vi "FTW-TestSupport-Reflection-TypeCoverage.vi"(0 "Types Tested":T1[](array[typedef]), 5 "Skip Types that cannot be instantiated":bool=TRUE, 11 "error in":errorcluster) -> (15 "error out":errorcluster)   [LabVIEW 2014]
uses:
  src/reflection/FTW-Reflection-Types.ctl
  src/error/FTW-ERR-ThrowError.vi
  src/error/FTW-ERR-NoErrorConstant.vi
  src/error/FTW-ERR-CallChain.vi
  src/string/FTW-STR-ReplaceWhitespace.vi
panel:
  # "Inputs"
  # "Outputs"
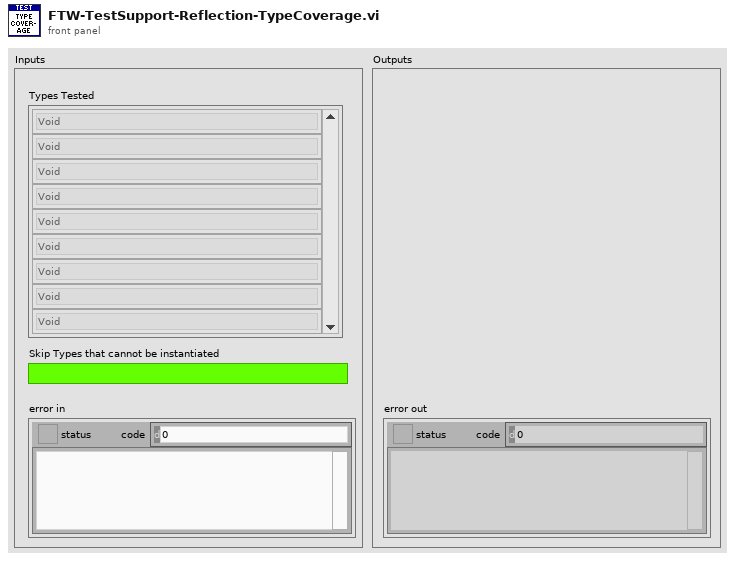
[diagram p1: front panel]
types:
  T1 = typedef "FTW-Reflection-Types.ctl" = enum16{"Unknown", "Void", "Array", "Cluster", "LVObject", "Boolean", "I8", "I16", "I32", "I64", "U8", "U16", "U32", "U64", "SGL", "DBL", "EXT", "CSG", "CDB", "CXT", "FXP", "EnumU8", "EnumU16", "EnumU32", "EnumU64", "SGLwithUnit", "DBLwithUnit", "EXTwithUnit", "CSGwithUnit", "CDBwithUnit", "CXTwithUnit", "String", "Path", "Picture", "Tag", "LVVariant", "Timestamp", "WaveformI8", "WaveformI16", "WaveformI32", "WaveformI64", "WaveformU8", "WaveformU16", "WaveformU32", "WaveformU64", "WaveformSGL", "WaveformDBL", "WaveformEXT", "WaveformCSG", "WaveformCDB", "WaveformCXT", "WaveformDigital", "WaveformUnknownType", "DigitalData", "DynamicData", "ExternalData", "FileByteStream", "TDMStream", "dotNET", "ActiveX", "VIServerReference", "VIReference", "ApplicationInstance", "Menu", "ConnectionDataSocket", "ConnectionVISA", "ConnectionBluetooth", "ConnectionIrDA", "ConnectionTCP", "ConnectionUDP", "ConnectionHTTPClient", "ConnectionFTP", "Occurrence", "Notifier", "Queue", "Rendezvous", "Semaphore", "RTFIFO", "EventPublisher", "EventRegistration", "EventCallback", "DataValueReference", "GenericClass", "GenericClassTag", "GenericClassDeepCopy", "GenericClassFlattened", "GenericClassTagFlattened", "GenericReferenceType", "WindowsRegistry", "OverloadedDatalogRef", "ReferenceUnknownType", "ByteArray", "ConPaneInterface"}
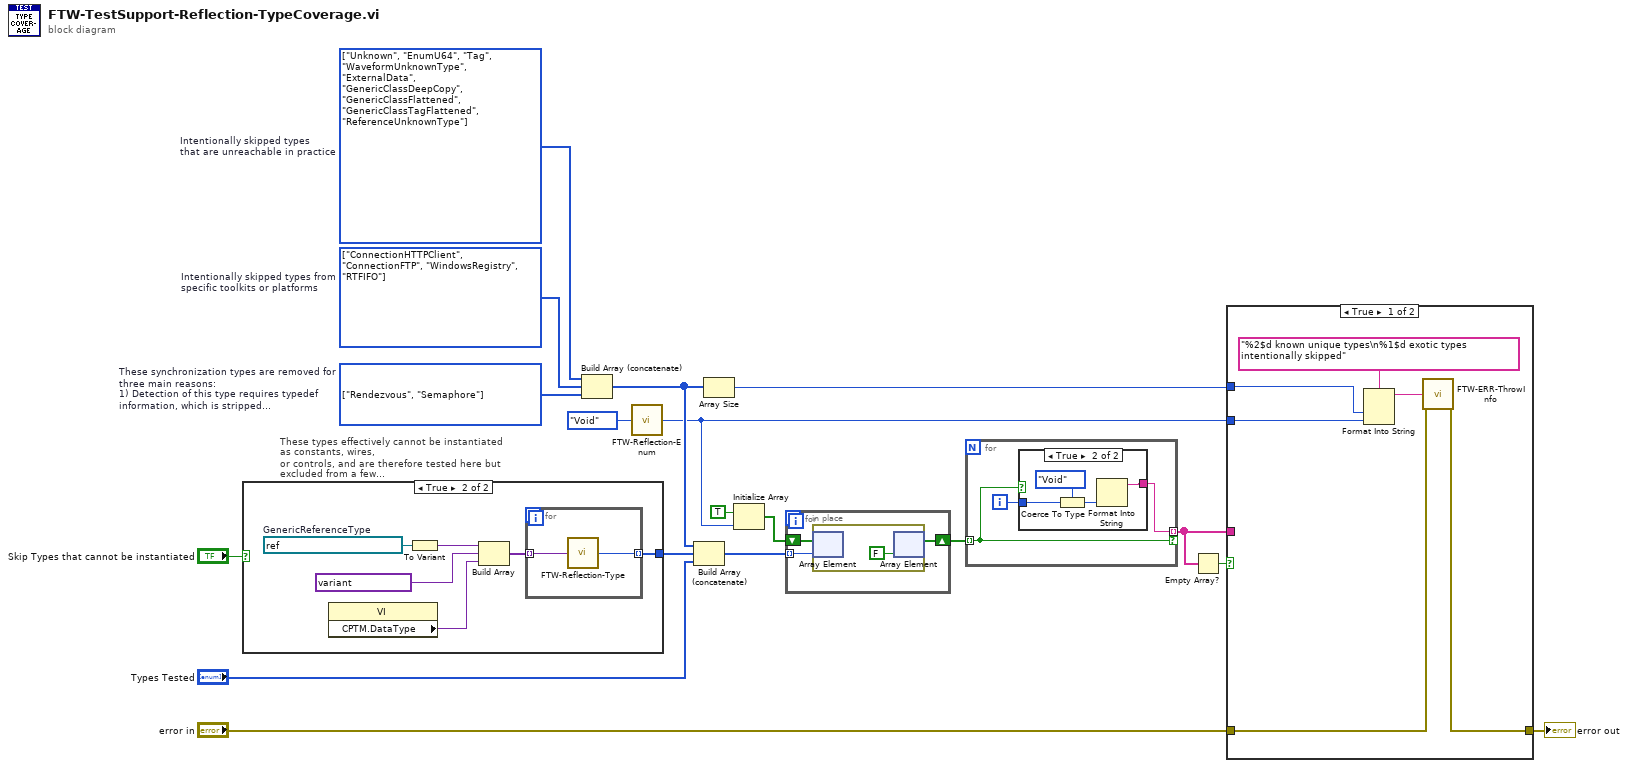
[diagram p0: block diagram]
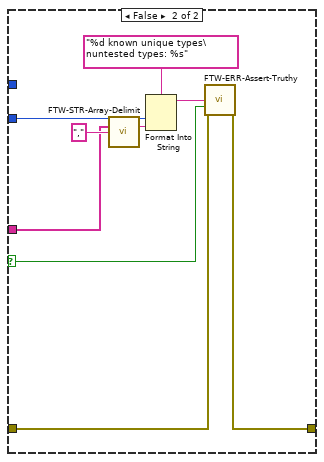
[diagram p2: hidden frame]
diagram:
  w1 = T1[] [enum."Rendezvous", enum."Semaphore"] items=["Unknown", "Void", "Array", "Cluster", "LVObject", "Boolean", "I8", "I16", "I32", "I64", "U8", "U16", "U32", "U64", "SGL", "DBL", "EXT", "CSG", "CDB", "CXT", "FXP", "EnumU8", "EnumU16", "EnumU32", "EnumU64", "SGLwithUnit", "DBLwithUnit", "EXTwithUnit", "CSGwithUnit", "CDBwithUnit", "CXTwithUnit", "String", "Path", "Picture", "Tag", "LVVariant", "Timestamp", "WaveformI8", "WaveformI16", "WaveformI32", "WaveformI64", "WaveformU8", "WaveformU16", "WaveformU32", "WaveformU64", "WaveformSGL", "WaveformDBL", "WaveformEXT", "WaveformCSG", "WaveformCDB", "WaveformCXT", "WaveformDigital", "WaveformUnknownType", "DigitalData", "DynamicData", "ExternalData", "FileByteStream", "TDMStream", "dotNET", "ActiveX", "VIServerReference", "VIReference", "ApplicationInstance", "Menu", "ConnectionDataSocket", "ConnectionVISA", "ConnectionBluetooth", "ConnectionIrDA", "ConnectionTCP", "ConnectionUDP", "ConnectionHTTPClient", "ConnectionFTP", "Occurrence", "Notifier", "Queue", "Rendezvous", "Semaphore", "RTFIFO", "EventPublisher", "EventRegistration", "EventCallback", "DataValueReference", "GenericClass", "GenericClassTag", "GenericClassDeepCopy", "GenericClassFlattened", "GenericClassTagFlattened", "GenericReferenceType", "WindowsRegistry", "OverloadedDatalogRef", "ReferenceUnknownType", "ByteArray", "ConPaneInterface"]  # These synchronization types are removed for three main reasons: 1) Detection of this type requires typedef information, which is stripped when this type is included in a container type (ConPane, Cluster ...) 2) These types likely are of negative value in an application, and have better alternatives 3) They are the last vestige linking FTW-Core directly to vi.lib
  w13 = T1[] [enum."ConnectionHTTPClient", enum."ConnectionFTP", enum."WindowsRegistry", enum."RTFIFO"] items=["Unknown", "Void", "Array", "Cluster", "LVObject", "Boolean", "I8", "I16", "I32", "I64", "U8", "U16", "U32", "U64", "SGL", "DBL", "EXT", "CSG", "CDB", "CXT", "FXP", "EnumU8", "EnumU16", "EnumU32", "EnumU64", "SGLwithUnit", "DBLwithUnit", "EXTwithUnit", "CSGwithUnit", "CDBwithUnit", "CXTwithUnit", "String", "Path", "Picture", "Tag", "LVVariant", "Timestamp", "WaveformI8", "WaveformI16", "WaveformI32", "WaveformI64", "WaveformU8", "WaveformU16", "WaveformU32", "WaveformU64", "WaveformSGL", "WaveformDBL", "WaveformEXT", "WaveformCSG", "WaveformCDB", "WaveformCXT", "WaveformDigital", "WaveformUnknownType", "DigitalData", "DynamicData", "ExternalData", "FileByteStream", "TDMStream", "dotNET", "ActiveX", "VIServerReference", "VIReference", "ApplicationInstance", "Menu", "ConnectionDataSocket", "ConnectionVISA", "ConnectionBluetooth", "ConnectionIrDA", "ConnectionTCP", "ConnectionUDP", "ConnectionHTTPClient", "ConnectionFTP", "Occurrence", "Notifier", "Queue", "Rendezvous", "Semaphore", "RTFIFO", "EventPublisher", "EventRegistration", "EventCallback", "DataValueReference", "GenericClass", "GenericClassTag", "GenericClassDeepCopy", "GenericClassFlattened", "GenericClassTagFlattened", "GenericReferenceType", "WindowsRegistry", "OverloadedDatalogRef", "ReferenceUnknownType", "ByteArray", "ConPaneInterface"]  # Intentionally skipped types from specific toolkits or platforms
  w14 = T1[] [enum."Unknown", enum."EnumU64", enum."Tag", enum."WaveformUnknownType", enum."ExternalData", enum."GenericClassDeepCopy", enum."GenericClassFlattened", enum."GenericClassTagFlattened", enum."ReferenceUnknownType"] items=["Unknown", "Void", "Array", "Cluster", "LVObject", "Boolean", "I8", "I16", "I32", "I64", "U8", "U16", "U32", "U64", "SGL", "DBL", "EXT", "CSG", "CDB", "CXT", "FXP", "EnumU8", "EnumU16", "EnumU32", "EnumU64", "SGLwithUnit", "DBLwithUnit", "EXTwithUnit", "CSGwithUnit", "CDBwithUnit", "CXTwithUnit", "String", "Path", "Picture", "Tag", "LVVariant", "Timestamp", "WaveformI8", "WaveformI16", "WaveformI32", "WaveformI64", "WaveformU8", "WaveformU16", "WaveformU32", "WaveformU64", "WaveformSGL", "WaveformDBL", "WaveformEXT", "WaveformCSG", "WaveformCDB", "WaveformCXT", "WaveformDigital", "WaveformUnknownType", "DigitalData", "DynamicData", "ExternalData", "FileByteStream", "TDMStream", "dotNET", "ActiveX", "VIServerReference", "VIReference", "ApplicationInstance", "Menu", "ConnectionDataSocket", "ConnectionVISA", "ConnectionBluetooth", "ConnectionIrDA", "ConnectionTCP", "ConnectionUDP", "ConnectionHTTPClient", "ConnectionFTP", "Occurrence", "Notifier", "Queue", "Rendezvous", "Semaphore", "RTFIFO", "EventPublisher", "EventRegistration", "EventCallback", "DataValueReference", "GenericClass", "GenericClassTag", "GenericClassDeepCopy", "GenericClassFlattened", "GenericClassTagFlattened", "GenericReferenceType", "WindowsRegistry", "OverloadedDatalogRef", "ReferenceUnknownType", "ByteArray", "ConPaneInterface"]  # Intentionally skipped types that are unreachable in practice
  n1 = case "These types effectively cannot be instantiated as constants, wires,\nor controls, and are therefore tested here but excluded from a few\ntypes of Reflection testing where it doesn't make sense" shown="True" "Skip Types that cannot be instantiated" {
    tunnel: [_ w19] -> w7
    frame False {
    }
    frame True {
      w21 = refnum<k0> refnum  # GenericReferenceType
      n2 = property class="VI"() -> ("CPTM.DataType"=w23:variant)  [unwired: 2 in, 2 out]
      n3 = To Variant(anything=w21) -> (Variant=w20:variant)
      n4 = Build Array(w20, variant, w23) -> (w22:variant[])
      n5 = for {
        tunnel: w22 -> [w26] mode=indexing
        tunnel: [w25] -> w19 mode=indexing
        n6 = call "FTW-Reflection-Type.vi"("Anything"=w26) -> ("LabVIEW Type"=w25:T1)  [unwired: 12 in, 2 out]
      }
    }
  }
  n7 = Build Array (concatenate)(w14, w13, w1) -> (w12:T1[])
  n8 = call "FTW-Reflection-Enum.vi"("Enum"=FTW-Reflection-Types."Void" ("y")) -> ("Number of Items"=w3:i32)  [unwired: 12 in, 2 out]
  n9 = Build Array (concatenate)(w12, w7, "Types Tested") -> (w11:T1[])
  n10 = Array Size(array=w12) -> (size(s)=w4:i32)
  n11 = Initialize Array(TRUE, w3) -> (w16:bool[])
  n12 = for {
    shift-right: [w28] -> w15
    shift-left: w16 -> [w29]
    tunnel: w11 -> [w27] mode=indexing
    n13 = in-place {
      n14 = in-place-array #1(w29, w27) -> ()  [unwired: 1 out]
      n15 = in-place-array #1(FALSE ("element")) -> (w28:bool[])  [unwired: 1 out]
    }
  }
  n16 = for {
    tunnel: w15 -> [w31] mode=indexing
    tunnel: [w32] -> w2 mode=indexing if=w31
    i -> [w33]
    n17 = case shown="True" w31 {
      tunnel: w33 -> [_ w37]
      tunnel: [_ w35] -> w32
      frame False {
      }
      frame True {
        n18 = Coerce To Type(0:w37, 1:FTW-Reflection-Types."Void" ("y")) -> (2:w36:T1)
        n19 = Format Into String(w36) -> (resulting string=w35:string)  [unwired: 3 in, 1 out]
      }
    }
  }
  n20 = Empty Array?(array=w2) -> (empty?=w5:bool)
  n21 = case shown="True" w5 {
    selector: w5 -> [_ w44]
    tunnel: [w43 w51] -> w9
    tunnel: "error in" -> [w42 w52]
    tunnel: w4 -> [w40 _]
    tunnel: w3 -> [w39 w47]
    tunnel: w2 -> [_ w49]
    frame True {
      n22 = Format Into String(format string="%2$d known unique types\n%1$d exotic types intentionally skipped", w40, w39) -> (resulting string=w38:string)  [unwired: 2 in, 1 out]
      n23 = call "FTW-ERR-ThrowInfo.vi"("Informational Message"=w38, "error in"=w42) -> ("error out"=w43:errorcluster)  [unwired: 13 in]
    }
    frame False {
      n24 = call "FTW-STR-Array-Delimit.vi"("Array of Strings"=w49, "Delimiter"=",") -> ("Delimited String"=w48:string)  [unwired: 13 in]
      n25 = Format Into String(format string="%d known unique types\nuntested types: %s", w47, w48) -> (resulting string=w45:string)  [unwired: 2 in, 1 out]
      n26 = call "FTW-ERR-Assert-Truthy.vi"("Assertion"=w45, "Assertion holds true?"=w44, "error in"=w52) -> ("error out"=w51:errorcluster)  [unwired: 12 in]
    }
  }
  "error out" <- w9
